vi "Init.vi"(10 "input":string[](array[string]), 11 "Volcano in":refnum<class "Volcano.lvclass">) -> (3 "Volcano out":refnum<class "Volcano.lvclass">)   [LabVIEW 2021, in "d16.lvlib" / "Volcano.lvclass"]
uses:
  Volcano.lvclass
  Volcano.lvclass/Volcano.ctl
  317e8209-662c-4c31-af41-99644d260e76.vi
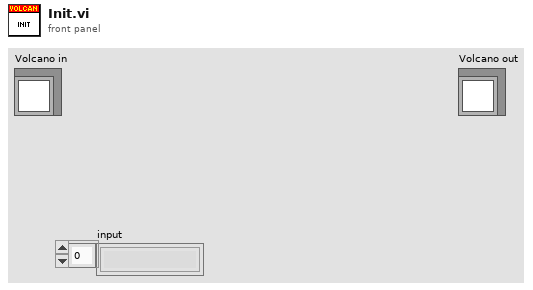
[diagram p1: front panel]
types:
  T1 = map{string, cluster{"Flow Rate":i32, "Routes":string[], "Route Time":i32[]}}
  T2 = cluster{"Current Valve":string, "Unopened Valves":string[], "Cumulative Pressure Released":u64, "Time":i32}
  T3 = cluster{"Flow Rate":i32, "Routes":string[], "Route Time":i32[]}
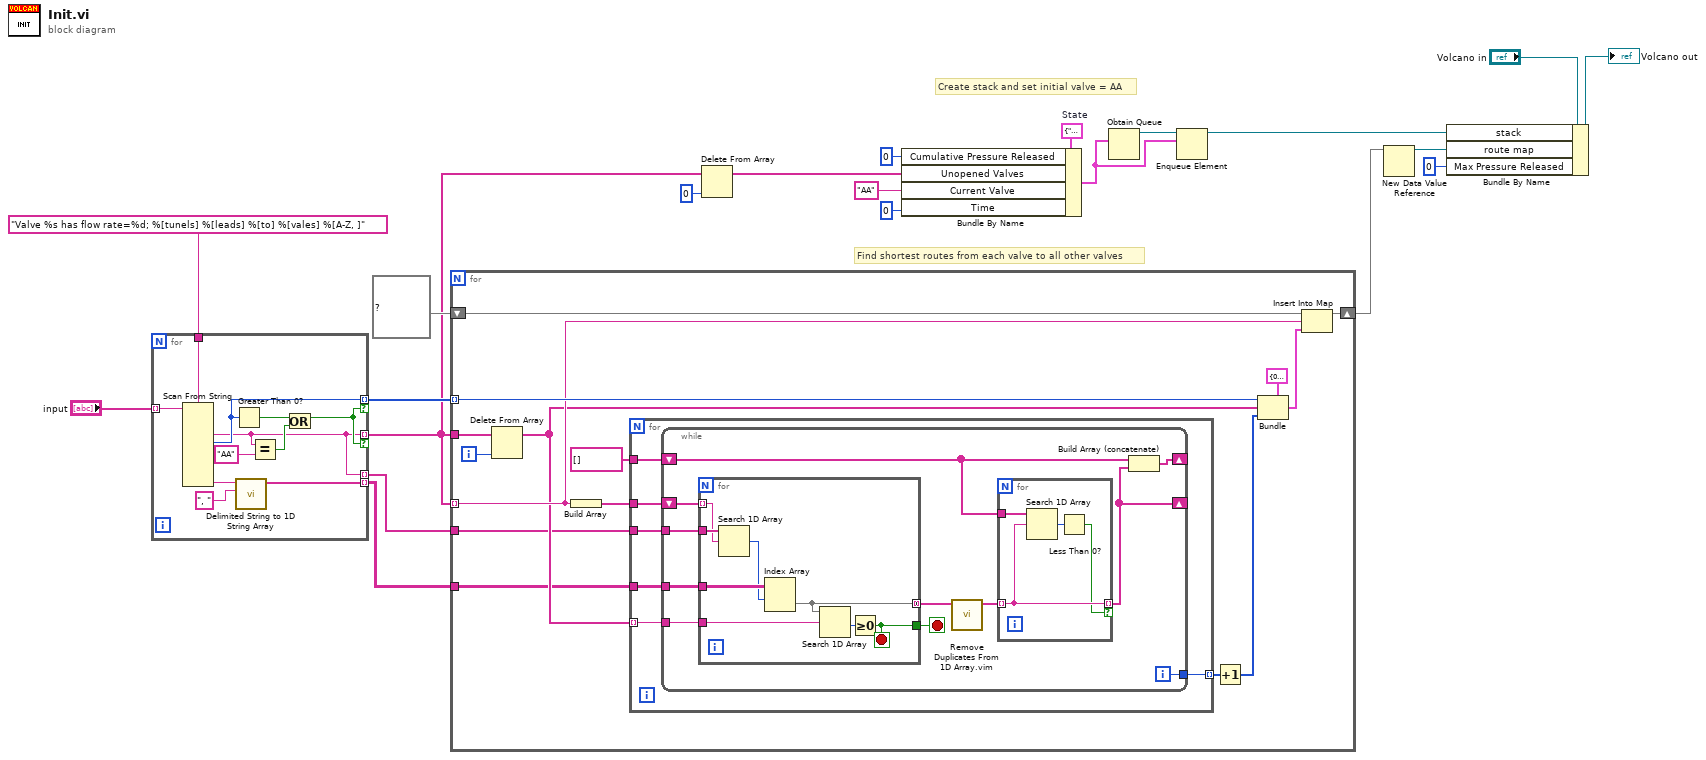
[diagram p0: block diagram]
diagram:
  w14 = T2 {"Current Valve"="AA", "Unopened Valves"=["AA"], "Cumulative Pressure Released"=0, "Time"=0}  # State
  # "Find shortest routes from each valve to all other valves"
  # "Create stack and set initial valve = AA"
  n1 = for {
    tunnel: "input" -> [w32] mode=indexing
    tunnel: "Valve %s has flow rate=%d; %[tunels] %[leads] %[to] %[vales] %[A-Z, ]" ("format string") -> [w31]
    tunnel: [w23] -> w3 mode=indexing if=w25
    tunnel: [w23] -> w19 mode=indexing
    tunnel: [w28] -> w18 mode=indexing if=w25
    tunnel: [w26] -> w17 mode=indexing
    n2 = Scan From String(format string=w31, input string=w32) -> (output 1=w23:string, output 2=w28:i32, output 7=w29:string)  [unwired: 13 in, 3 out]
    n3 = Greater Than 0?(x=w28) -> (x > 0?=w27:bool)
    n4 = call <vilib>:"Delimited String to 1D String Array.vi"("delimiter"=", ", "delimited string"=w29) -> ("string array"=w26:string[])  [unwired: 9 in]
    n5 = Equal?(x=w23, y="AA") -> (x = y?=w24:bool)
    n6 = Or(x=w27, y=w24) -> (x .or. y?=w25:bool)
  }
  n7 = for {
    tunnel: w19 -> [w39]
    tunnel: w3 -> [w41] mode=indexing
    tunnel: w3 -> [w45]
    shift-right: [w47] -> w6
    shift-left: T1 {} ("map out") -> [w46]
    tunnel: w18 -> [w43] mode=indexing
    tunnel: w17 -> [w38]
    i -> [w44]
    n8 = Delete From Array(array=w45, index=w44) -> (array with subset deleted=w40:string[])  [unwired: 1 in, 1 out]
    n9 = Build Array(w41) -> (w37:string[])
    n10 = for {
      tunnel: w40 -> [w53] mode=indexing
      tunnel: w39 -> [w52]
      tunnel: w38 -> [w51]
      tunnel: w37 -> [w50]
      tunnel: [w49] -> w36 mode=indexing
      tunnel: string[] [] -> [w48]
      n11 = while {
        tunnel: w53 -> [w62]
        tunnel: w52 -> [w64]
        shift-right: [w54] -> _
        shift-left: w50 -> [w59]
        tunnel: [w61] -> w49
        shift-right: [w55] -> _
        shift-left: w48 -> [w56]
        tunnel: w51 -> [w63]
        i -> [w61]
        stop <- w60 stop-if-true
        n12 = for {
          tunnel: w64 -> [w76]
          tunnel: w59 -> [w69] mode=indexing
          tunnel: w63 -> [w75]
          tunnel: [w73] -> w58 mode=concatenating
          tunnel: w62 -> [w72]
          tunnel: [w70] -> w60
          stop <- w70 stop-if-true
          n13 = Search 1D Array(1D array=w76, element=w69) -> (index of element=w74:i32)  [unwired: 1 in]
          n14 = Index Array(array=w75, index (row)=w74) -> (element=w73:string[])  [unwired: 1 in]
          n15 = Search 1D Array(1D array=w73, element=w72) -> (index of element=w71:i32)  [unwired: 1 in]
          n16 = Greater Or Equal To 0?(x=w71) -> (x >= 0?=w70:bool)
        }
        n17 = call "Remove Duplicates From 1D Array.vim"("array"=w58) -> ("array with duplicates removed"=w57:string[])  [unwired: 10 in]
        n18 = for {
          tunnel: w57 -> [w67] mode=indexing
          tunnel: w56 -> [w68]
          tunnel: [w67] -> w54 mode=indexing if=w65
          n19 = Search 1D Array(1D array=w68, element=w67) -> (index of element=w66:i32)  [unwired: 1 in]
          n20 = Less Than 0?(x=w66) -> (x < 0?=w65:bool)
        }
        n21 = Build Array (concatenate)(w56, w54) -> (w55:string[])
      }
    }
    n22 = Increment(x=w36) -> (x+1=w35:i32[])
    n23 = Bundle(cluster=T3 {"Flow Rate"=0, "Routes"=[], "Route Time"=[]}, "Flow Rate"=w43, "Routes"=w40, "Route Time"=w35) -> (w42:T3)
    n24 = Insert Into Map(map in=w46, key=w41, value=w42) -> (map out=w47:T1)  [unwired: 2 out]
  }
  n25 = Delete From Array(array=w3, index=0) -> (array with subset deleted=w1:string[])  [unwired: 1 in, 1 out]
  n26 = Bundle By Name(cluster=w14, "Cumulative Pressure Released"=u64 0, "Unopened Valves"=w1, "Current Valve"="AA", "Time"=0) -> (w11:T2)
  n27 = Obtain Queue(element data type=w11) -> (queue out=w12:refnum<queue>)  [unwired: 4 in, 2 out]
  n28 = Enqueue Element(queue=w12, element=w11) -> (queue out=w4:refnum<queue>)  [unwired: 2 in, 2 out]
  n29 = New Data Value Reference(data value=w6) -> (data value reference=w9:refnum<data-value>)  [unwired: 1 in, 1 out]
  n30 = Bundle By Name(cluster="Volcano in", "stack"=w4, "route map"=w9, "Max Pressure Released"=u64 0) -> (→"Volcano out":refnum<class "Volcano.lvclass">)
